vi "氨氮测量数据储存.vi"   [LabVIEW 2016, in "斯坦道氨氮.lvlib"]
types:
  T1 = cluster{"时间标识":timestamp, "测量模式":enum16{"维护数据", "水样测试", "标样核查", "零点核查", "跨度核查", "空白测试", "平行样测试", "加标回收", "空白校准", "标样校准", "初始化（清洗）"}, "数据标记表":string, "监测值":sgl, "单位":u16, "数据标识":string, "因子编码":u32, "标样参考值":sgl, "F0":sgl, "F1":sgl, "F2":sgl, "F3":sgl, "F4":sgl, "F5":sgl, "F6":sgl, "F7":sgl, "X":sgl, "温度":sgl, "湿度":sgl, "量程标识":string, "SN":string}
  T2 = enum16{"维护数据", "水样测试", "标样核查", "零点核查", "跨度核查", "空白测试", "平行样测试", "加标回收", "空白校准", "标样校准", "初始化（清洗）"}
  T3 = cluster{"系统时间":timestamp, "工作状态":enum16{"空闲", "水样测试", "标样核查", "零点核查", "跨度核查", "空白测试", "平行样测试", "加标回收", "空白校准", "标样校准", "初始化（清洗）"}, "测量模式":enum16{"待机", "连续模式", "周期模式", "定点模式", "受控模式", "手动模式"}, "告警代码":u16, "故障代码":u16, "日志代码":u16, "软件版本":u16, "F0":sgl, "F1":sgl, "F2":sgl, "F3":sgl, "T":sgl, "H":sgl, "id":u16, "flowid":u16, "量程":u16, "总磷控温温度1":sgl, "营养盐控温温度2":sgl, "ADC":sgl}
  T4 = cluster{"运行模式":enum16{"维护模式", "常规模式", "应急模式", "质控模式"}, "质控频次":enum16{"关闭", "每天", "星期一", "星期二", "星期三", "星期四", "星期五", "星期六", "星期日"}, "空白核查时间":u16, "跨度核查时间":u16, "24H周期设置":bool[]}
  T5 = enum16{"空闲", "水样测试", "标样核查", "零点核查", "跨度核查", "空白测试", "平行样测试", "加标回收", "空白校准", "标样校准", "初始化（清洗）"}
  T6 = cluster{"因子编码":u32, "单位":u16, "标样参考值":sgl, "水样数据时间":timestamp, "水样实测值":sgl, "水样数据标识":string, "标样数据时间":timestamp, "标样实测值":sgl, "标样数据标识":string, "空白数据时间":timestamp, "空白实测值":sgl, "空白数据标识":string, "零点核查数据时间":timestamp, "零点核查实测值":sgl, "零点核查数据标识":string, "跨度核查数据时间":timestamp, "跨度核查实测值":sgl, "跨度核查数据标识":string, "加标回收数据时间":timestamp, "加标回收实测值":sgl, "加标回收数据标识":string, "平行样数据时间":timestamp, "平行样实测值":sgl, "平行样数据标识":string, "F0":sgl, "F1":sgl, "F2":sgl, "F3":sgl, "F4":sgl, "F5":sgl, "F6":sgl, "F7":sgl, "温度":sgl, "湿度":sgl, "X值":sgl}
  T7 = cluster{"氨氮跨度值":dbl, "氨氮零点标准液浓度":dbl, "氨氮跨度标准液浓度":dbl, "氨氮标准液标准浓度":dbl}
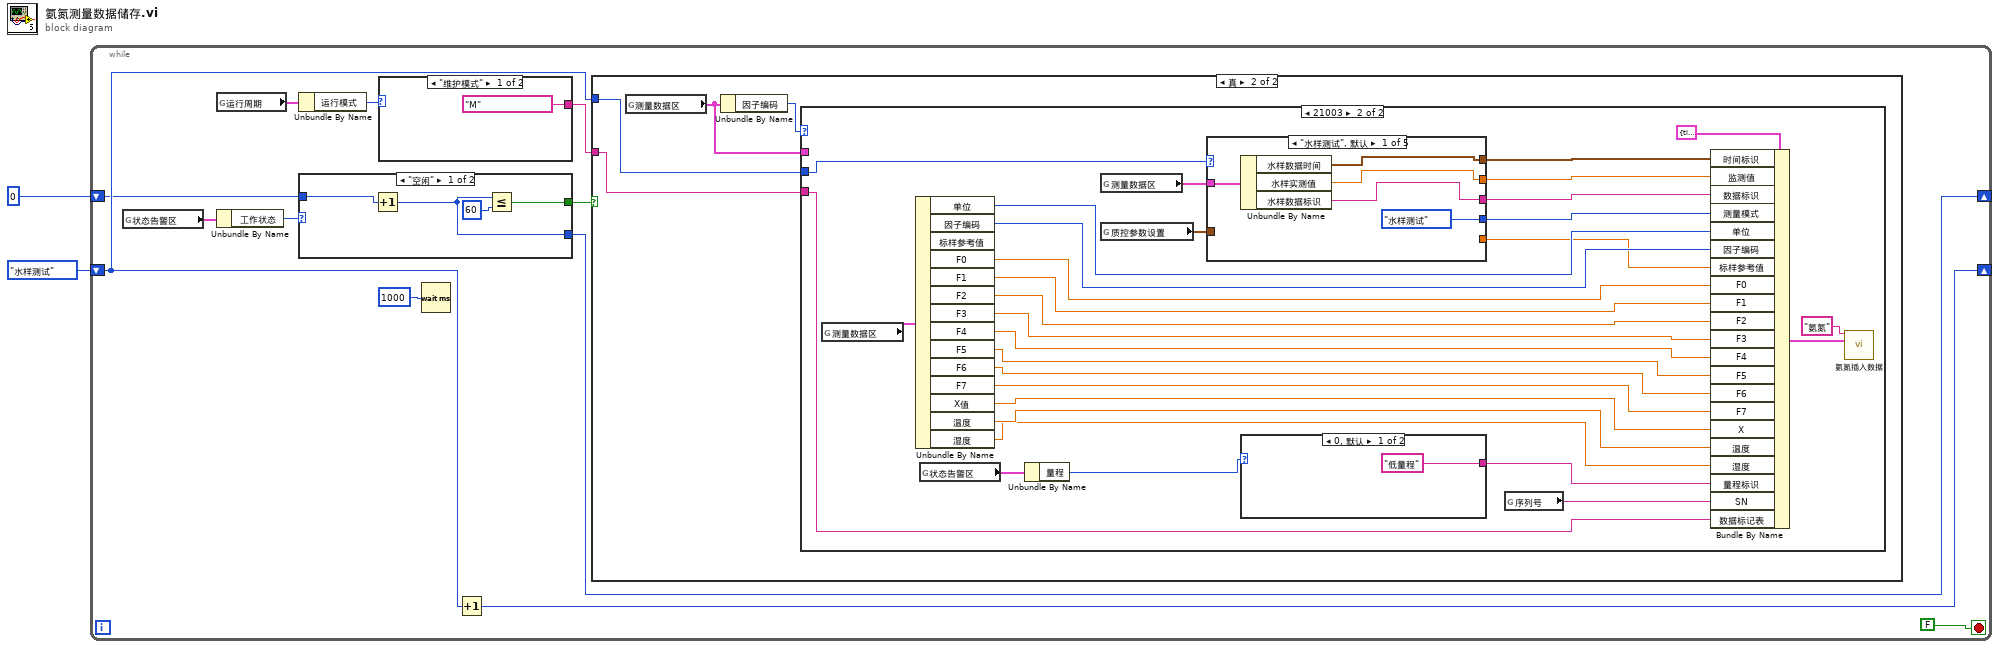
[diagram p0: block diagram]
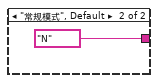
[diagram p3: hidden frame]
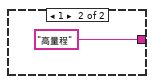
[diagram p6: hidden frame]
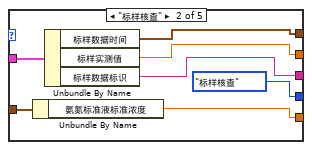
[diagram p7: hidden frame]
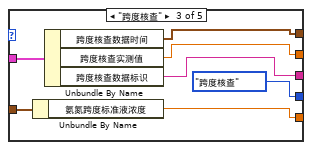
[diagram p8: hidden frame]
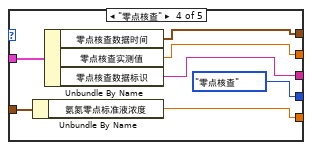
[diagram p9: hidden frame]
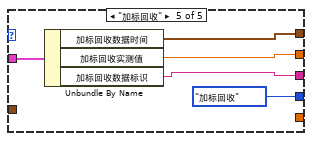
[diagram p10: hidden frame]
diagram:
  n1 = while {
    shift-right: [w11] -> _
    shift-left: enum16{"水样测试", "标样核查", "跨度核查", "零点核查", "加标回收"}."水样测试" ("测量模式") -> [w10]
    shift-right: [w4] -> _
    shift-left: u32 0 ("等待时间（毫秒）") -> [w5]
    stop <- FALSE stop-if-true
    n2 = global read "VAR氨氮全局变量.vi" "状态告警区"() -> (w7:T3)
    n3 = global read "氨氮断电保存全局变量.vi" "运行周期"() -> (w9:T4)
    n4 = Unbundle By Name(w7) -> ("工作状态"=w6:T5)
    n5 = Unbundle By Name(w9) -> ("运行模式"=w8:enum16{"维护模式", "常规模式", "应急模式", "质控模式"})
    n6 = case shown="\"空闲\"" w6 {
      tunnel: w5 -> [w18 _]
      tunnel: [w17 _] -> w4
      tunnel: [w15 _] -> w3
      frame "空闲" {
        n7 = Increment(x=w18) -> (x+1=w17:u32)
        n8 = Less Or Equal?(x=w17, y=u32 60) -> (x <= y?=w15:bool)
      }
      frame "水样测试", Default {
      }
    }
    n9 = case shown="\"维护模式\"" w8 {
      tunnel: ["M" ("数据标记表") "N" ("数据标记表")] -> w12
      frame "维护模式" {
      }
      frame "常规模式", Default {
      }
    }
    n10 = Wait (ms)(milliseconds to wait=u32 1000 ("等待时间（毫秒）")) -> ()  [unwired: 1 out]
    n11 = Increment(x=w10) -> (x+1=w11:enum16{"水样测试", "标样核查", "跨度核查", "零点核查", "加标回收"})
    n12 = case shown="真" w3 {
      tunnel: w12 -> [_ w22]
      tunnel: w10 -> [_ w21]
      frame False {
      }
      frame True {
        n13 = global read "VAR氨氮全局变量.vi" "测量数据区"() -> (w24:T6)
        n14 = Unbundle By Name(w24) -> ("因子编码"=w23:u32)
        n15 = case shown="21003" w23 {
          tunnel: w24 -> [_ _]
          tunnel: w22 -> [_ w27]
          tunnel: w21 -> [_ w38]
          frame Default {
          }
          frame 21003 {
            n16 = global read "VAR氨氮全局变量.vi" "测量数据区"() -> (w41:T6)
            n17 = Unbundle By Name(w41) -> ("单位"=w53:u16, "因子编码"=w52:u32, "F0"=w51:sgl, "F1"=w50:sgl, "F2"=w49:sgl, "F3"=w48:sgl, "F4"=w47:sgl, "F5"=w46:sgl, "F6"=w45:sgl, "F7"=w44:sgl, "X值"=w34:sgl, "温度"=w43:sgl, "湿度"=w42:sgl)  [unwired: 1 out]
            n18 = global read "VAR氨氮全局变量.vi" "状态告警区"() -> (w26:T3)
            n19 = Unbundle By Name(w26) -> ("量程"=w25:u16)
            n20 = global read "VAR氨氮全局变量.vi" "测量数据区"() -> (w54:T6)
            n21 = global read "氨氮断电保存全局变量.vi" "质控参数设置"() -> (w37:T7)
            n22 = case shown="\"水样测试\", 默认" w38 {
              tunnel: w54 -> [w61 w68 w75 w82 w87]
              tunnel: [w60 w67 w74 w81 w86] -> w33
              tunnel: [w59 w66 w73 w80 w85] -> w39
              tunnel: [w58 w65 w72 w79 w84] -> w40
              tunnel: [T2."水样测试" ("测量模式") T2."标样核查" ("测量模式") T2."跨度核查" ("测量模式") T2."零点核查" ("测量模式") T2."加标回收" ("测量模式")] -> w28
              tunnel: w37 -> [_ w63 w70 w77 _]
              tunnel: [_ w62 w69 w76 _] -> w36
              frame "水样测试", Default {
                n23 = Unbundle By Name(w61) -> ("水样数据时间"=w60:timestamp, "水样实测值"=w59:sgl, "水样数据标识"=w58:string)
              }
              frame "标样核查" {
                n24 = Unbundle By Name(w63) -> ("氨氮标准液标准浓度"=w62:dbl)
                n25 = Unbundle By Name(w68) -> ("标样数据时间"=w67:timestamp, "标样实测值"=w66:sgl, "标样数据标识"=w65:string)
              }
              frame "跨度核查" {
                n26 = Unbundle By Name(w70) -> ("氨氮跨度标准液浓度"=w69:dbl)
                n27 = Unbundle By Name(w75) -> ("跨度核查数据时间"=w74:timestamp, "跨度核查实测值"=w73:sgl, "跨度核查数据标识"=w72:string)
              }
              frame "零点核查" {
                n28 = Unbundle By Name(w77) -> ("氨氮零点标准液浓度"=w76:dbl)
                n29 = Unbundle By Name(w82) -> ("零点核查数据时间"=w81:timestamp, "零点核查实测值"=w80:sgl, "零点核查数据标识"=w79:string)
              }
              frame "加标回收" {
                n30 = Unbundle By Name(w87) -> ("加标回收数据时间"=w86:timestamp, "加标回收实测值"=w85:sgl, "加标回收数据标识"=w84:string)
              }
            }
            n31 = case shown="0, 默认" w25 {
              tunnel: ["低量程" ("database") "高量程" ("database")] -> w35
              frame 0, Default {
              }
              frame 1 {
              }
            }
            n32 = global read "VAR氨氮全局变量.vi" "序列号"() -> (w29:string)
            n33 = Bundle By Name(cluster=T1 {"时间标识"=timestamp(0 s since 1904-01-01), "测量模式"=enum."水样测试", "数据标记表"="N", "监测值"=0.0, "单位"=0, "数据标识"="", "因子编码"=0, "标样参考值"=0.0, "F0"=0.0, "F1"=0.0, "F2"=0.0, "F3"=0.0, "F4"=0.0, "F5"=0.0, "F6"=0.0, "F7"=0.0, "X"=0.0, "温度"=0.0, "湿度"=0.0, "量程标识"="", "SN"=""} ("data"), "时间标识"=w33, "监测值"=w39, "数据标识"=w40, "测量模式"=w28, "单位"=w53, "因子编码"=w52, "标样参考值"=w36, "F0"=w51, "F1"=w50, "F2"=w49, "F3"=w48, "F4"=w47, "F5"=w46, "F6"=w45, "F7"=w44, "X"=w34, "温度"=w43, "湿度"=w42, "量程标识"=w35, "SN"=w29, "数据标记表"=w27) -> (w30:T1)
            n34 = call "氨氮插入数据.vi"("table"="氨氮", "data"=w30) -> ()  [unwired: 13 in, 1 out]
          }
        }
      }
    }
  }
